vi "ParseCommand.vi"(0 "Command string":string) -> (1 "Command":string, 2 "Parameters":string[](array[string]))   [LabVIEW 2015]
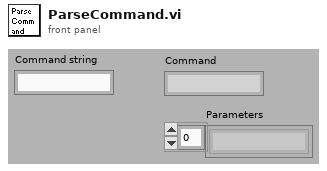
[diagram p1: front panel]
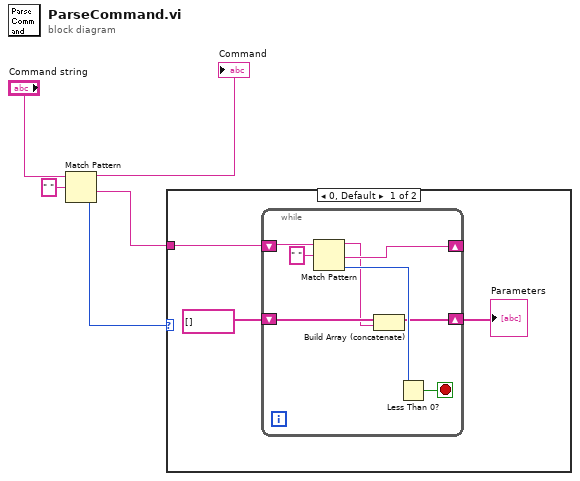
[diagram p0: block diagram]
diagram:
  n1 = Match Pattern(string="Command string", regular expression=" ") -> (before substring=→"Command":string, after substring=w2:string, offset past match=w1:i32)  [unwired: 1 in, 1 out]
  n2 = case shown="0, Default" w1 {
    tunnel: w2 -> [w7 _]
    frame 0, Default {
      n3 = while {
        shift-right: [w12] -> _
        shift-left: w7 -> [w16]
        shift-right: [w9] -> w6
        shift-left: string[] [] -> [w11]
        stop <- w13 stop-if-true
        n4 = Match Pattern(string=w16, regular expression=" ") -> (before substring=w10:string, after substring=w12:string, offset past match=w14:i32)  [unwired: 1 in, 1 out]
        n5 = Build Array (concatenate)(w11, w10) -> (w9:string[])
        n6 = Less Than 0?(x=w14) -> (x < 0?=w13:bool)
      }
      "Parameters" <- w6
    }
    frame -1 {
    }
  }
